vi "MagnetoGUI.vi"() -> ()   [LabVIEW 2016]
panel:
  out "faktor 2":dbl
  out "faktor 1":dbl
  out "theoretische Primaerwindungszahl":dbl
  in  "Gwuenschte Frequenz [Hz]":dbl=15.0 min=15.0 max=15000.0 step=5.0
  in  "Gewuenschte magn. Flussdichte [T]":dbl=0.001 min=0.001 max=5.0 step=0.001
  in  "Messwiderstand [Ohm]":dbl=1.0 min=1.0 max=100.0
  in  "Spannungsteilerverhaeltnis (1/x)":dbl=1.0 min=1.0 max=100.0 step=1.0
  in  "Sekundaerwindungszahl":dbl=1.0 min=1.0 max=1500.0 step=1.0
  in  "Primaerwindungszahl":dbl=1.0 min=1.0 max=1500.0 step=1.0
  in  "Dichte des Eisens in [g/cm^3]":dbl=1.0 min=1.0 max=50.0 step=1.0
  in  "Eisenquerschnitt A [mm^2]":dbl=1.0 min=1.0 max=10000.0 step=1.0
  in  "Wirksame Laenge [cm]":dbl=94.0 min=0.0001 max=1000.0 step=0.5
  in  "Probenbezeichnung":string
  # "Eingabe-Parameter"
  # "z.B. 94"
  # "Berechnete Konstanten"
  # "z.B. 45"
  # "z.B. 7"
  # "z.B. 700"
  # "z.B. 700"
  # "z.B. 1"
  # "z.B. 1"
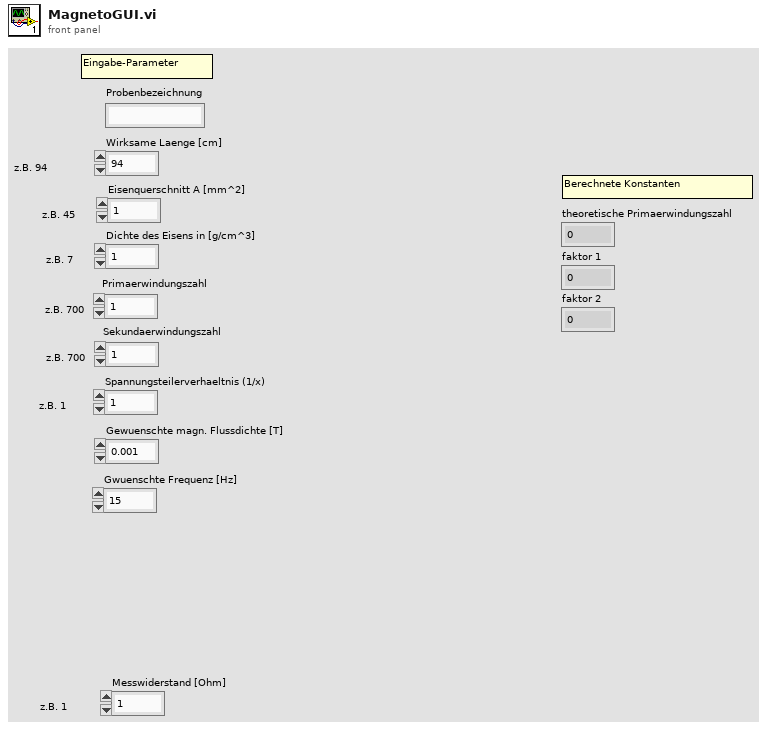
[diagram p1: front panel]
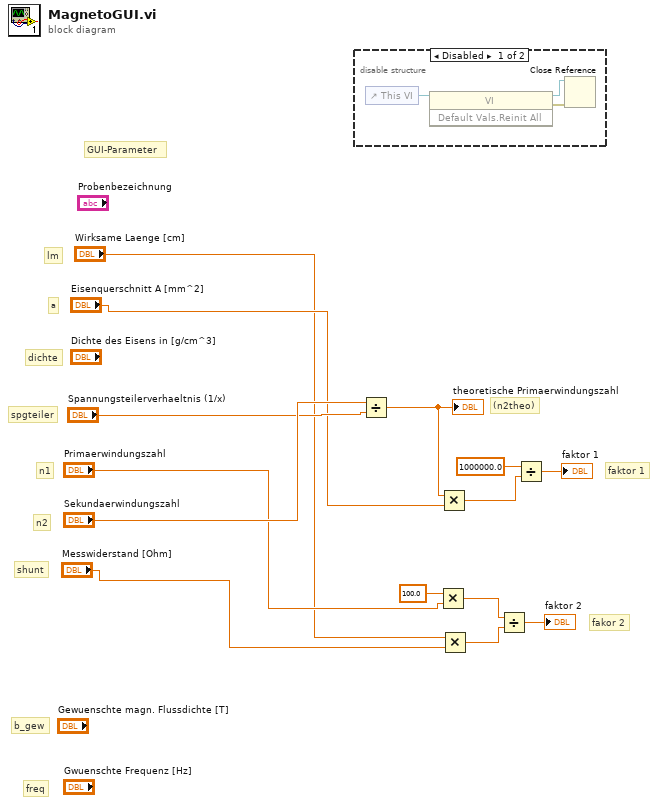
[diagram p0: block diagram]
diagram:
  # "freq"
  # "b_gew"
  # "fakor 2"
  # "faktor 1"
  # "spgteiler"
  # "dichte"
  # "shunt"
  # "n2"
  # "n1"
  # "a"
  # "lm"
  # "(n2theo)"
  # "GUI-Parameter"
  n1 = disable-structure shown="Disabled" {
    frame Disabled {
      n2 = control-ref of="This VI"() -> (w17:refnum<vi>)
      n3 = invoke class="VI" method="Default Vals.Reinit All"(reference=w17) -> (reference out=w16:refnum<vi>, error out=w15:errorcluster)  [unwired: 2 in, 1 out]
      n4 = Close Reference(reference=w16, error in (no error)=w15) -> ()  [unwired: 1 out]
    }
    frame Enabled {
    }
  }
  n5 = Divide(x="Sekundaerwindungszahl", y="Spannungsteilerverhaeltnis (1/x)") -> (x/y=w11:dbl)
  "theoretische Primaerwindungszahl" <- w11
  n6 = Multiply(x=100.0, y="Primaerwindungszahl") -> (x*y=w2:dbl)
  n7 = Multiply(x=w11, y="Eisenquerschnitt A [mm^2]") -> (x*y=w10:dbl)
  n8 = Multiply(x="Wirksame Laenge [cm]", y="Messwiderstand [Ohm]") -> (x*y=w3:dbl)
  n9 = Divide(x=w2, y=w3) -> (x/y=→"faktor 2":dbl)
  n10 = Divide(x=1000000.0, y=w10) -> (x/y=→"faktor 1":dbl)
